vi "WindowMotorValue.vi"() -> ()   [LabVIEW 2016]
panel:
  out "WindowMotorValue":dbl
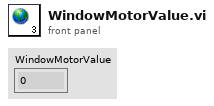
[diagram p1: front panel]
diagram:
